vi "Load Config.vi"(6 "Constants":refnum<class "Sequence Constants.lvclass">, 8 "error in (no error)":refnum<class "MultiErrors.lvclass">, 10 "Config Element":refnum<class "Config Element.lvclass">, 11 "Set Var Command Config in":refnum<class "Set Var Command Config.lvclass">) -> (0 "error out":refnum<class "MultiErrors.lvclass">, 3 "Set Var Command Config out":refnum<class "Set Var Command Config.lvclass">)   [LabVIEW 2020, in "VolatusSeqConfig.lvlib" / "Set Var Command Config.lvclass"]
uses:
  Set Var Command Config.lvclass
  VolatusErrorUtilities/MultiErrors/MultiErrors.lvclass
  lv-cdm/CDM-Config/Config Element/Config Element.lvclass
  Sequence Constants/Sequence Constants.lvclass
  Set Var Command Config.lvclass/Set Var Command Config.ctl
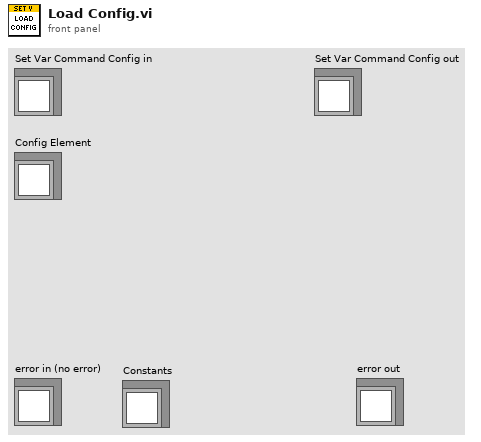
[diagram p1: front panel]
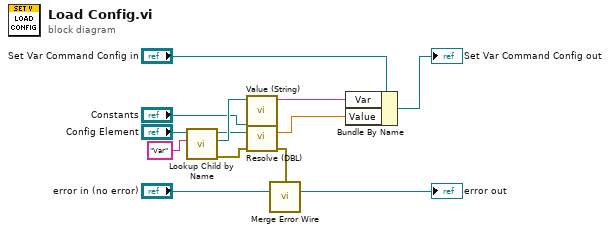
[diagram p0: block diagram]
diagram:
  n1 = call "Lookup Child by Name.vi"("Name"="Var", "Config Element in"="Config Element") -> ("error out"=w4:errorcluster, "Child"=w13:refnum<class "Config Element.lvclass">, "Config Element out"=w5:refnum<class "Config Element.lvclass">)  [unwired: 6 in, 1 out]
  n2 = call "Value (String).vi"("Config Element in"=w13) -> ("String Value"=w12:string)  [unwired: 9 in, 1 out]
  n3 = call "Resolve (DBL).vi"("error in (no error)"=w4, "Element"=w5, "Sequence Constants in"="Constants") -> ("error out"=w3:errorcluster, "DBL Value"=w2:dbl)  [unwired: 6 in, 1 out]
  n4 = call "Merge Error Wire.vi"("error in (no error)"=w3, "MultiErrors in"="error in (no error)") -> ("MultiErrors out"=→"error out":refnum<class "MultiErrors.lvclass">)  [unwired: 13 in]
  n5 = Bundle By Name(cluster="Set Var Command Config in", "Var"=w12, "Value"=w2) -> (→"Set Var Command Config out":refnum<class "Set Var Command Config.lvclass">)
